vi "Bullet Markdown.vi"(8 "error in":errorcluster, 11 "File Path":path) -> (0 "error out":errorcluster, 2 "Wiki entry":string, 3 "Rendered metadata":string)   [LabVIEW 2021]
panel:
  out "result string":string
  out "String":string
  out "first subarray":string[](array[string])
  out "group/channel names":string[][](array[string])
  out "property values":variant[](array[variant])
  out "property names":string[](array[string])
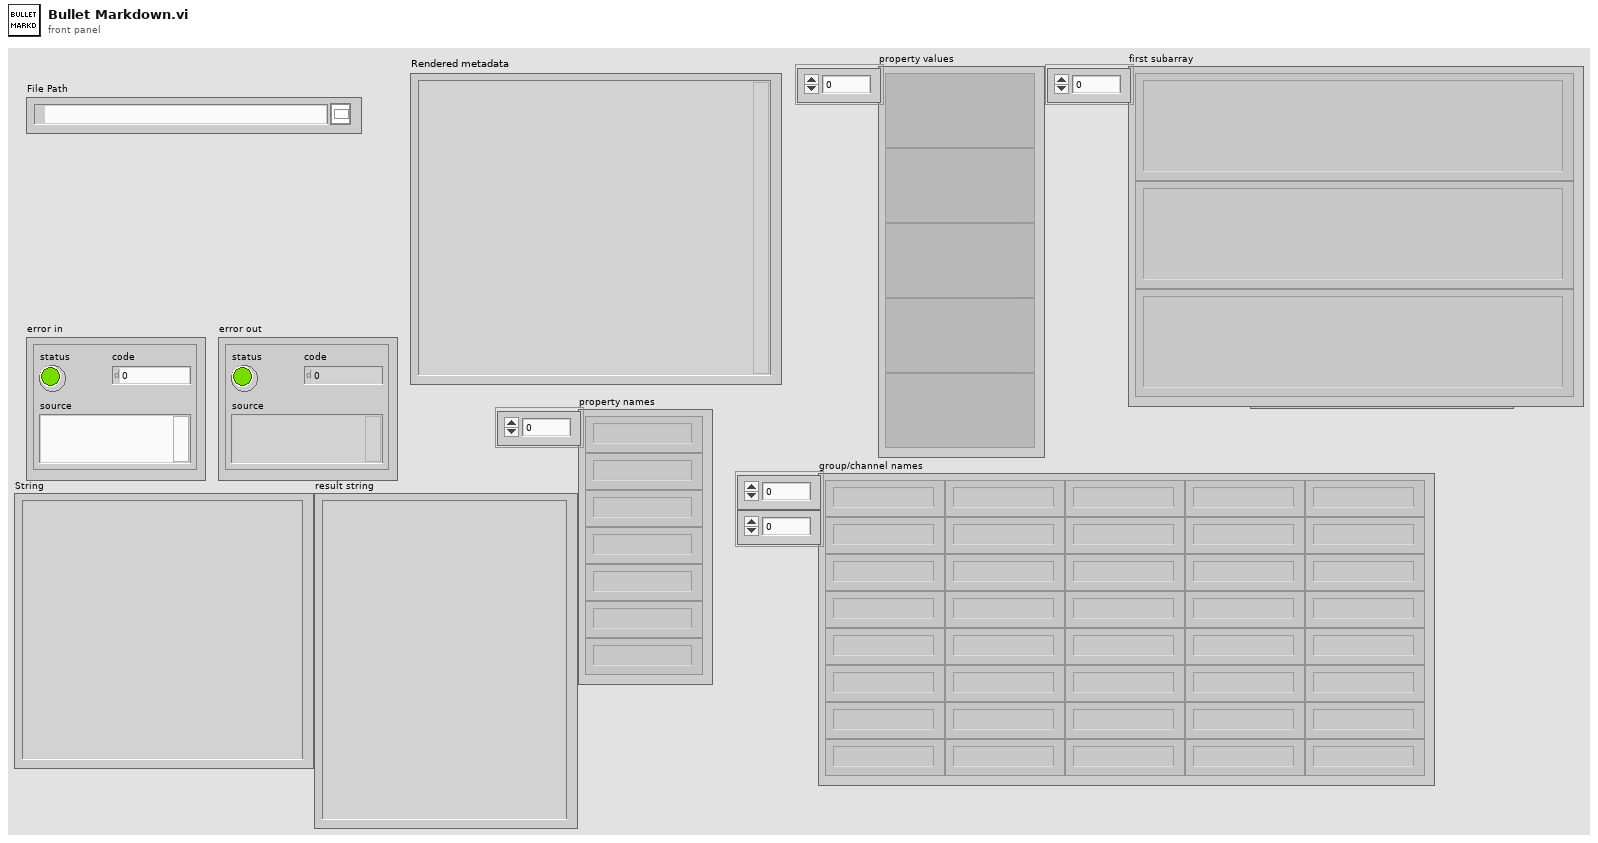
[diagram p1: front panel]
types:
  T1 = enum16{"open", "open or create", "create or replace", "create", "open (read-only)"}
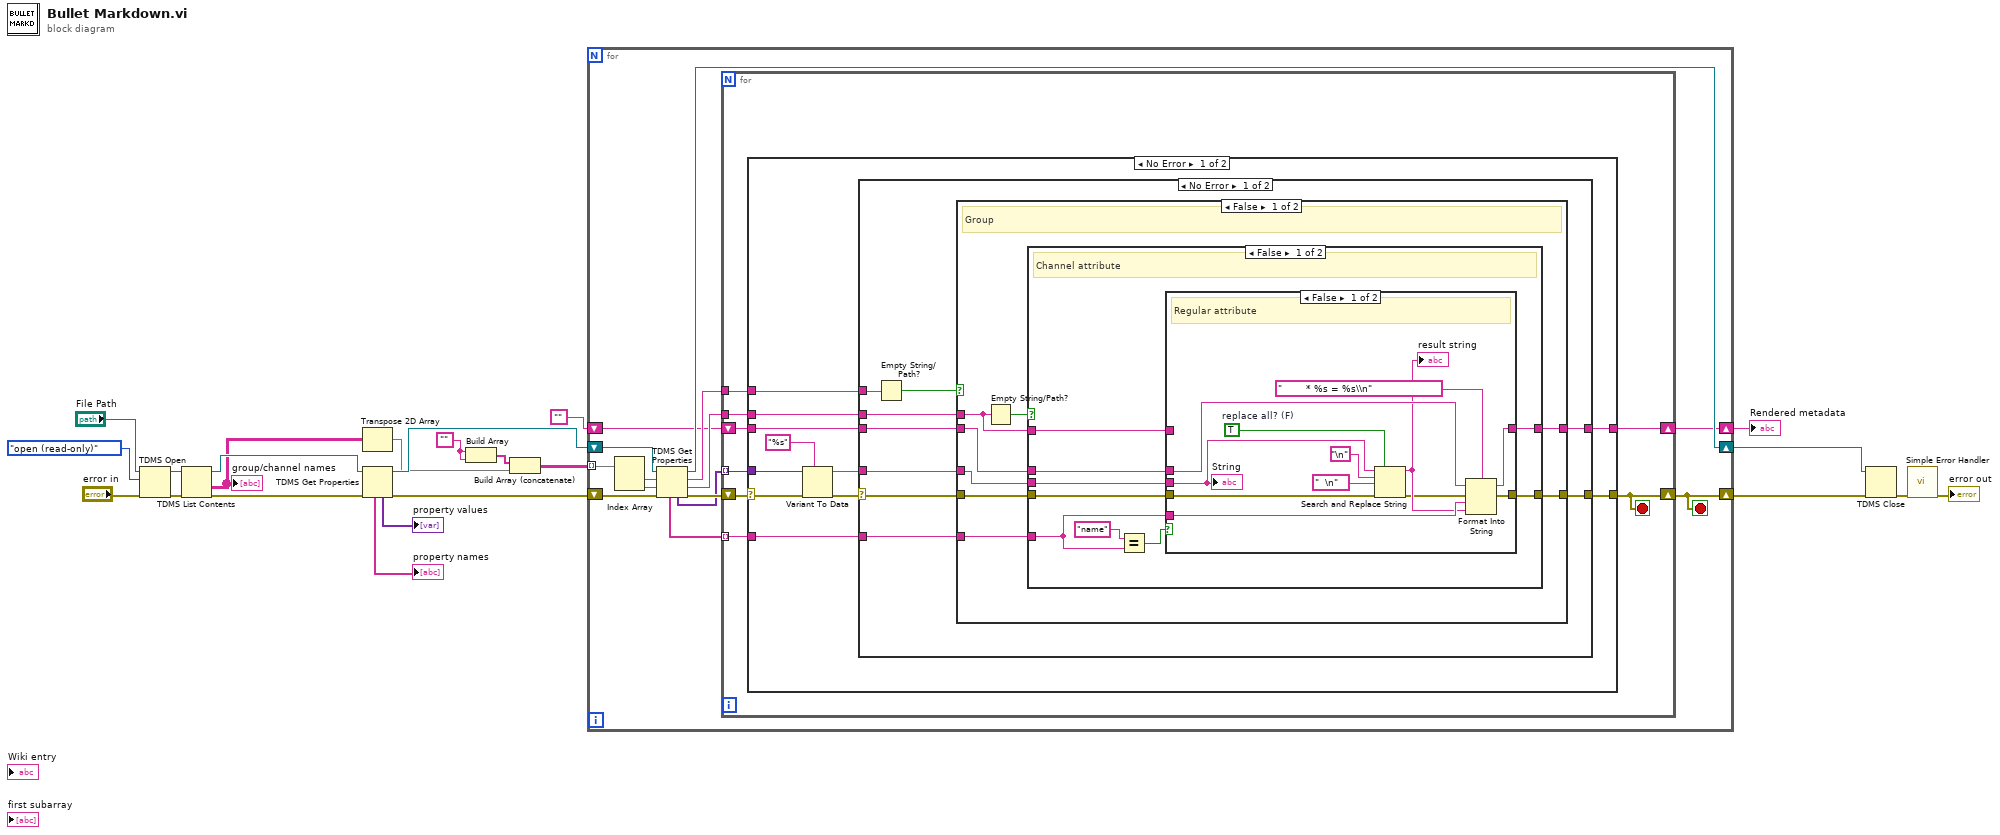
[diagram p0: block diagram]
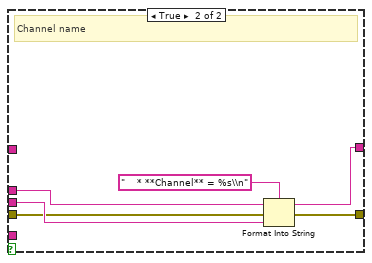
[diagram p2: hidden frame]
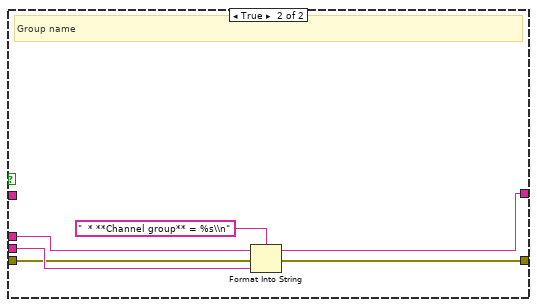
[diagram p3: hidden frame]
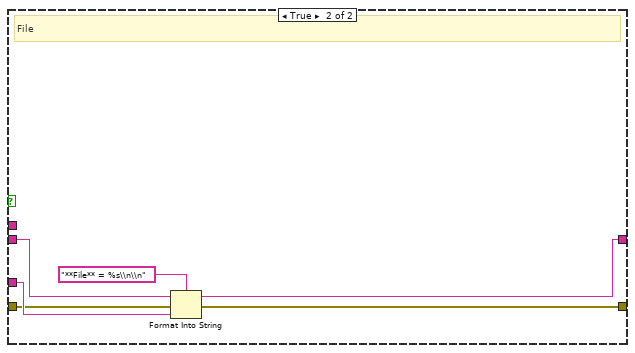
[diagram p4: hidden frame]
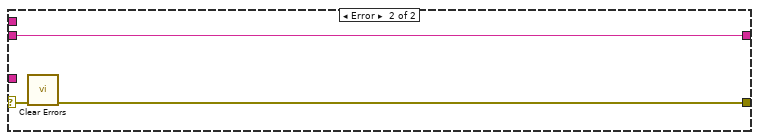
[diagram p5: hidden frame]
diagram:
  w5 = ""
  n1 = TDMS Open(8:"error in", 10:T1."open (read-only)" ("operation (0:open)"), 11:"File Path") -> (0:w16:errorcluster, 3:w14:refnum<k34>)  [unwired: 4 in]
  n2 = TDMS List Contents(4:w16, 7:w14) -> (0:w15:errorcluster, 1:w3:string[][], 3:w13:refnum<k34>)  [unwired: 1 in, 1 out]
  "group/channel names" <- w3
  n3 = Transpose 2D Array(2D array=w3) -> (transposed array=w2:string[][])
  n4 = TDMS Get Properties(8:w15, 11:w13) -> (0:w11:errorcluster, 3:w12:refnum<k34>, 4:→"property values":variant[], 6:→"property names":string[])  [unwired: 4 in, 2 out]
  n5 = Build Array(w5, w5) -> (w4:string[])
  n6 = Build Array (concatenate)(w4, w2) -> (w1:string[][])
  n7 = for {
    tunnel: w1 -> [w36] mode=indexing
    shift-right: [w31] -> w10
    shift-left: w12 -> [w33]
    shift-right: [w23] -> w9
    shift-left: w11 -> [w32]
    shift-right: [w25] -> w7
    shift-left: "" -> [w26]
    stop <- w23 stop-if-true
    n8 = Index Array(array=w36) -> (element #1=w35:string, element #2=w34:string)  [unwired: 2 in]
    n9 = TDMS Get Properties(8:w32, 9:w34, 10:w35, 11:w33) -> (0:w28:errorcluster, 1:w29:string, 2:w30:string, 3:w31:refnum<k34>, 4:w24:variant[], 6:w27:string[])  [unwired: 2 in]
    n10 = for {
      tunnel: w30 -> [w44]
      tunnel: w29 -> [w43]
      tunnel: w27 -> [w42] mode=indexing
      shift-right: [w38] -> w23
      shift-left: w28 -> [w39]
      shift-right: [w37] -> w25
      shift-left: w26 -> [w41]
      tunnel: w24 -> [w40] mode=indexing
      stop <- w38 stop-if-true
      n11 = case shown="No Error" w39 {
        selector: w39 -> [w45 w116]
        tunnel: w44 -> [w55 _]
        tunnel: w43 -> [w54 _]
        tunnel: [w53 w116] -> w38
        tunnel: w42 -> [w52 _]
        tunnel: w41 -> [w51 w115]
        tunnel: [w50 w115] -> w37
        tunnel: w40 -> [w49 _]
        frame No Error {
          n12 = Variant To Data(error in=w45, type="%s", Variant=w49) -> (data=w47:string, error out=w46:errorcluster)
          n13 = case shown="No Error" w46 {
            selector: w46 -> [w56 w113]
            tunnel: w55 -> [w64 _]
            tunnel: w54 -> [w59 _]
            tunnel: [w57 w112] -> w53
            tunnel: w52 -> [w58 _]
            tunnel: w51 -> [w62 w114]
            tunnel: [w60 w114] -> w50
            tunnel: w47 -> [w61 _]
            frame No Error {
              n14 = Empty String/Path?(string/path=w64) -> (empty?=w63:bool)
              n15 = case shown="False" w63 {
                tunnel: w62 -> [w71 w110]
                tunnel: w61 -> [w70 w111]
                tunnel: [w69 w108] -> w60
                tunnel: w59 -> [w68 _]
                tunnel: w58 -> [w67 _]
                tunnel: [w66 w107] -> w57
                tunnel: w56 -> [w65 w106]
                frame False {
                  # "Group"
                  n16 = Empty String/Path?(string/path=w68) -> (empty?=w72:bool)
                  n17 = case shown="False" w72 {
                    tunnel: w71 -> [w81 w104]
                    tunnel: w70 -> [w79 w103]
                    tunnel: [w78 w102] -> w69
                    tunnel: w68 -> [w80 _]
                    tunnel: w67 -> [w77 _]
                    tunnel: [w74 w101] -> w66
                    tunnel: w65 -> [w73 w100]
                    frame False {
                      # "Channel attribute"
                      n18 = Equal?(x="name", y=w77) -> (x = y?=w75:bool)
                      n19 = case shown="False" w75 {
                        tunnel: w81 -> [w92 w98]
                        tunnel: w80 -> [_ _]
                        tunnel: w77 -> [w91 _]
                        tunnel: w79 -> [w89 w96]
                        tunnel: [w90 w97] -> w78
                        tunnel: [w83 w95] -> w74
                        tunnel: w73 -> [w82 w94]
                        frame False {
                          w85 = TRUE  # replace all? (F)
                          # "Regular attribute"
                          n20 = Search and Replace String(replace all?=w85, input string=w89, search string="\n", replace string="  \n" ("replace string (\"\")"), error in=w82) -> (result string=w88:string, error out=w84:errorcluster)  [unwired: 3 in, 2 out]
                          "result string" <- w88
                          n21 = Format Into String(format string="        * %s = %s\\n", initial string=w92, error in=w84, w91, w88) -> (resulting string=w90:string, error out=w83:errorcluster)
                          "String" <- w89
                        }
                        frame True {
                          # "Channel name"
                          n22 = Format Into String(format string="    * **Channel** = %s\\n", initial string=w98, error in=w94, w96) -> (resulting string=w97:string, error out=w95:errorcluster)
                        }
                      }
                    }
                    frame True {
                      # "Group name"
                      n23 = Format Into String(format string="  * **Channel group** = %s\\n", initial string=w104, error in=w100, w103) -> (resulting string=w102:string, error out=w101:errorcluster)
                    }
                  }
                }
                frame True {
                  # "File"
                  n24 = Format Into String(format string="**File** = %s\\n\\n", initial string=w110, error in=w106, w111) -> (resulting string=w108:string, error out=w107:errorcluster)
                }
              }
            }
            frame Error {
              n25 = call <vilib>:"Clear Errors.vi"("error in (no error)"=w113) -> ("error out"=w112:errorcluster)  [unwired: 5 in, 1 out]
            }
          }
        }
        frame Error {
        }
      }
    }
  }
  "Rendered metadata" <- w7
  n26 = TDMS Close(8:w9, 11:w10) -> (0:w19:errorcluster)  [unwired: 1 out]
  n27 = call <vilib>:"Simple Error Handler.vi"("error in (no error)"=w19) -> ("error out"=→"error out":errorcluster)  [unwired: 4 in, 4 out]
